vi "get publishers.vi"(8 "error in (no error)":errorcluster, 11 "manager_daemon in":refnum<class "manager_daemon.lvclass">) -> (0 "error out":errorcluster, 2 "Publisher Map":T1, 3 "manager_daemon out":refnum<class "manager_daemon.lvclass">)   [LabVIEW 2024, in "manager_daemon.lvclass"]
uses:
  manager_daemon.lvclass
  type_defs/PublisherMap--map.ctl
  type_defs/PublisherData--cluster.ctl
  type_defs/msg--cluster.ctl
  type_defs/cmd--enum.ctl
  manager_daemon.lvclass/manager_daemon.ctl
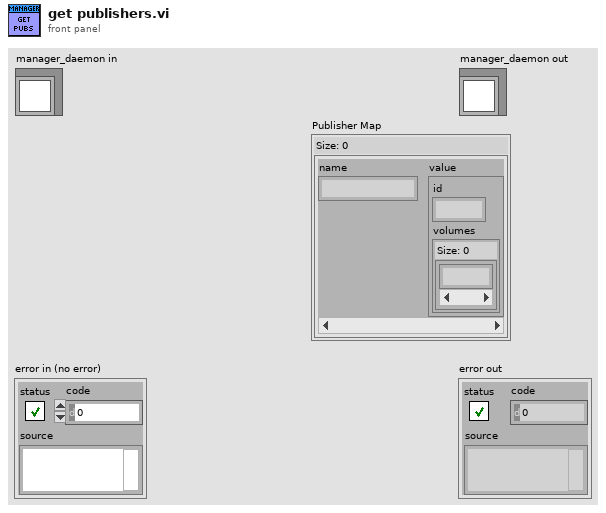
[diagram p1: front panel]
types:
  T1 = typedef "manager_daemon.lvclass/PublisherMap--map.ctl" = map{string, T2}
  T2 = typedef "manager_daemon.lvclass/PublisherData--cluster.ctl" = cluster{"id":i32, "volumes":set{i32}}
  T3 = typedef "manager_daemon.lvclass/cmd--enum.ctl" = enum16{"init", "run", "load binaries", "save binaries", "updated volume", "get set names", "return vol path by id", "return vol ids by publisher", "display info", "filter release week", "apply filter", "add publisher", "get publishers", "add volume", "add volumes", "add issues", "add issue", "delete volume", "delete issues", "download issues", "scan for reprints", "exit"}
  T4 = typedef "manager_daemon.lvclass/msg--cluster.ctl" = cluster{"cmd":T3, "data":variant}
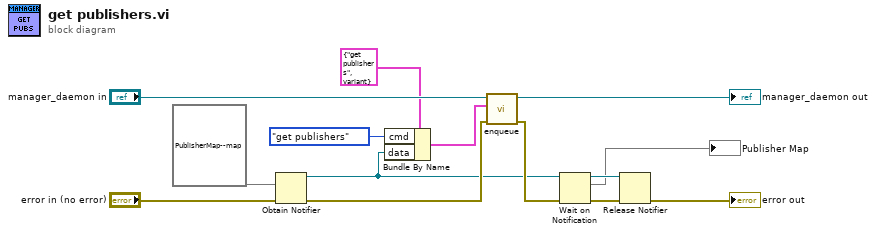
[diagram p0: block diagram]
diagram:
  n1 = Obtain Notifier(notification data type=T1 {} ("map"), error in (no error)="error in (no error)") -> (notifier out=w3:refnum<notifier>, error out=w11:errorcluster)  [unwired: 2 in, 1 out]
  n2 = Bundle By Name(cluster=T4 {"cmd"=enum."get publishers", "data"=variant} ("msg"), "cmd"=cmd--enum."get publishers", "data"=w3) -> (w1:T4)
  n3 = call "enqueue.vi"("error in (no error)"=w11, "msg"=w1, "manager_daemon in"="manager_daemon in") -> ("error out"=w10:errorcluster, "manager_daemon out"=→"manager_daemon out":refnum<class "manager_daemon.lvclass">)  [unwired: 7 in]
  n4 = Wait on Notification(notifier=w3, error in (no error)=w10) -> (notifier out=w7:refnum<notifier>, notification=→"Publisher Map":T1, error out=w8:errorcluster)  [unwired: 2 in, 1 out]
  n5 = Release Notifier(notifier=w7, error in (no error)=w8) -> (error out=→"error out":errorcluster)  [unwired: 1 in, 2 out]
